vi "Proceed.vi"(7 "component is ready (Y)":bool=TRUE, 8 "error in (no error)":errorcluster, 10 "ProceedMessage":refnum<class "ProceedMessage.lvclass">, 11 "MeritFactor in":refnum<class "MeritFactor.lvclass">) -> (0 "error out":errorcluster, 2 "all observers are ready?":bool, 3 "MeritFactor out":refnum<class "MeritFactor.lvclass">)   [LabVIEW 2012, in "MeritFactor.lvclass"]
uses:
  MeritFactor.lvclass
  <vilib>/Distrio/Murmex/ProceedMessage/ProceedMessage.lvclass
  <vilib>/Distrio/Murmex/Murmex/Murmex.lvclass
panel:
  # "This method is called when the PROCEED\ntrigger is sent. \n\nOverride this method when your component needs to\nrespond to this trigger. \n\nCall parent for proper implementation"
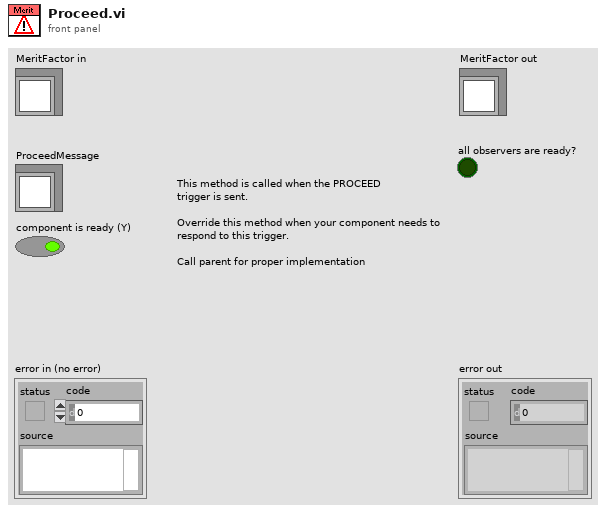
[diagram p1: front panel]
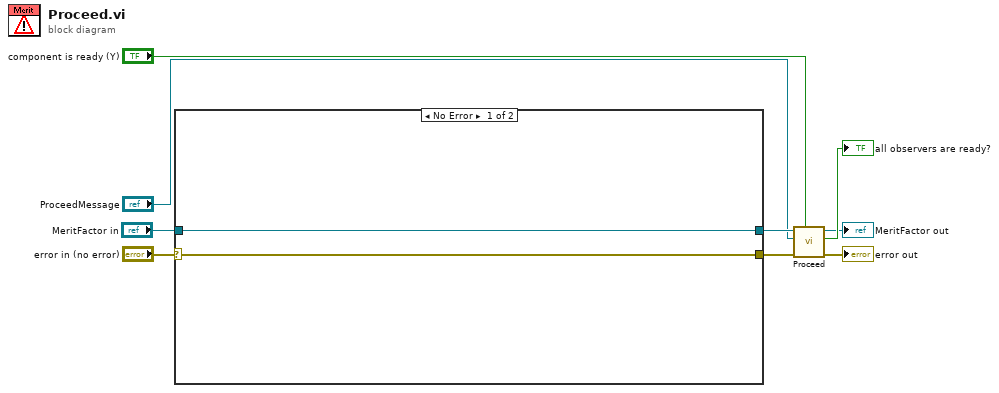
[diagram p0: block diagram]
diagram:
  n1 = case shown="No Error" "error in (no error)" {
    selector: "error in (no error)" -> [w11 w12]
    tunnel: "MeritFactor in" -> [w10 w13]
    tunnel: [w11 w12] -> w3
    tunnel: [w10 w13] -> w2
    frame No Error {
    }
    frame Error {
    }
  }
  n2 = call-parent "Proceed.vi"("component is ready (Y)"="component is ready (Y)", "error in (no error)"=w3, "ProceedMessage"="ProceedMessage", "Murmex in"=w2) -> ("error out"=→"error out":errorcluster, "all observers are ready?"=→"all observers are ready?":bool, "Murmex out"=→"MeritFactor out":refnum<class "MeritFactor.lvclass">)  [unwired: 5 in]
